vi "Script Cluster from JSON.vi"(6 "Update Values":bool, 8 "Error In":errorcluster, 10 "JSON String":string, 11 "VI Path":path) -> (0 "Errror Out":errorcluster)   [LabVIEW 2019, in "SLL JSON to Cluster.lvlib"]
doc: "This VI converts input JSON string to its equivalent cluster control in new VI"
uses:
  SLL JSON to Cluster.lvlib
  <vilib>/Utility/error.llb/Error Cluster From Error Code.vi
  <vilib>/ErrorRing/Error Ring.xnode
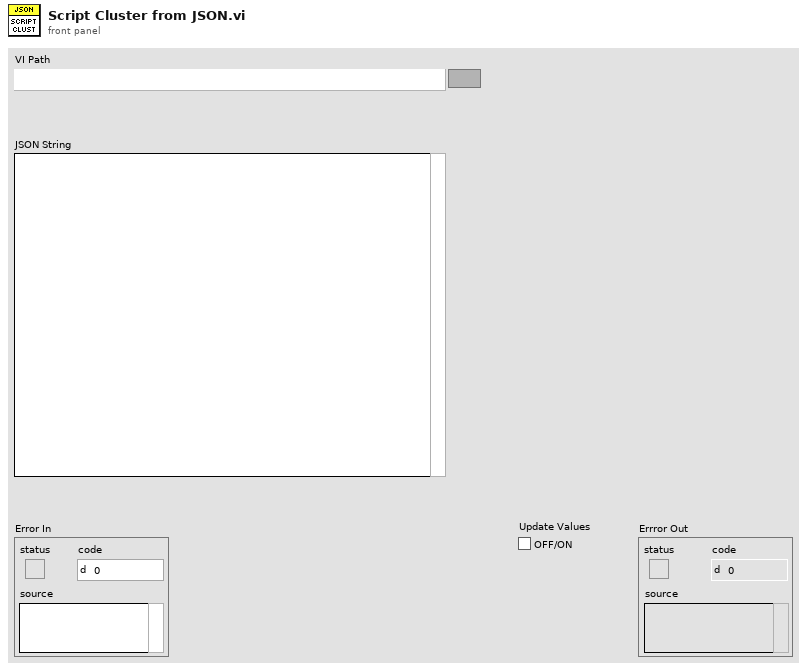
[diagram p1: front panel]
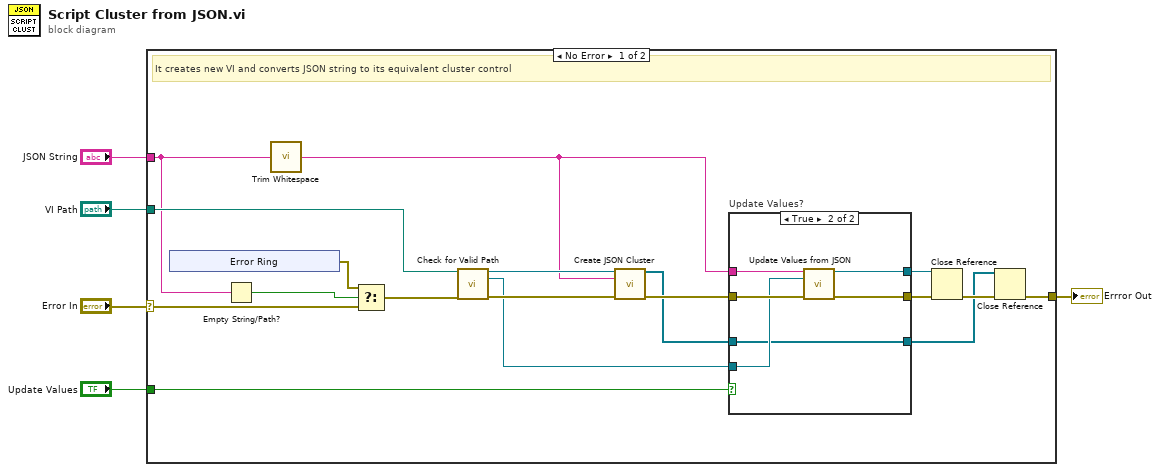
[diagram p0: block diagram]
diagram:
  n1 = case shown="No Error" "Error In" {
    selector: "Error In" -> [w22 w38]
    tunnel: [w20 w38] -> w4
    tunnel: "JSON String" -> [w16 _]
    tunnel: "VI Path" -> [w17 _]
    tunnel: "Update Values" -> [w8 _]
    frame No Error {
      # "It creates new VI and converts JSON string to its equivalent cluster control"
      n2 = xnode "Error Ring"() -> ("error out"=w21:errorcluster)
      n3 = Empty String/Path?(string/path=w16) -> (empty?=w23:bool)
      n4 = call <vilib>:"Trim Whitespace.vi"("string"=w16) -> ("trimmed string"=w13:string)  [unwired: 1 in]
      n5 = Select(t=w21, s=w23, f=w22) -> (s? t:f=w19:errorcluster)
      n6 = call "Check for Valid Path.vi"("Input VI Path"=w17, "Error In"=w19) -> ("Front Panel Reference"=w15:refnum<vi>, "VI Reference Out"=w12:refnum<vi>, "Error Out"=w18:errorcluster)  [unwired: 11 in]
      n7 = call "Create JSON Cluster.vi"("Front Panel Ref In"=w15, "JSON String"=w13, "Error In"=w18) -> ("Parent Ref Out"=w7:refnum<vi>[], "Error Out"=w14:errorcluster)  [unwired: 11 in]
      n8 = case "Update Values?" shown="True" w8 {
        tunnel: w14 -> [w25 w32]
        tunnel: w13 -> [_ w31]
        tunnel: w12 -> [w26 w30]
        tunnel: [w25 w29] -> w11
        tunnel: [w26 w28] -> w9
        tunnel: w7 -> [w24 w27]
        tunnel: [w24 w27] -> w6
        frame False {
        }
        frame True {
          n9 = call "Update Values from JSON.vi"("JSON String"=w31, "VI Ref In"=w30, "Error In"=w32) -> ("VI Ref Out"=w28:refnum<vi>, "Error Out"=w29:errorcluster)  [unwired: 11 in]
        }
      }
      n10 = Close Reference(reference=w9, error in (no error)=w11) -> (error out=w10:errorcluster)
      n11 = Close Reference(reference=w6, error in (no error)=w10) -> (error out=w20:errorcluster)
    }
    frame Error {
      # "If error, this case pass that error message"
    }
  }
  "Errror Out" <- w4
